vi "GFITS_GetLastHdrs.vi"(10 "ext":string) -> (2 "hdrs":string)   [LabVIEW 2016]
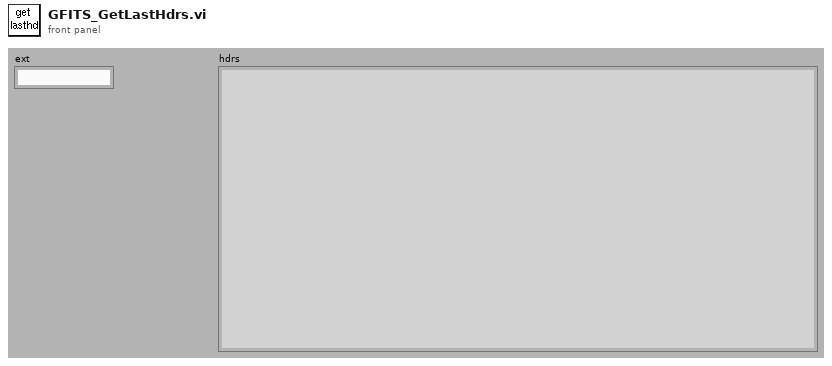
[diagram p1: front panel]
types:
  T1 = enum16{"clear all", "add extension", "add keyword", "get", "clear extension", "done"}
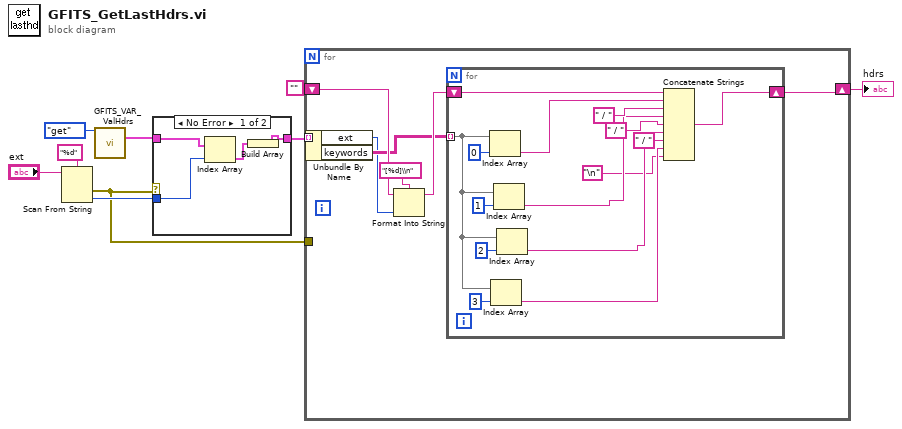
[diagram p0: block diagram]
diagram:
  n1 = Scan From String(format string="%d", input string="ext") -> (error out=w3:errorcluster, output 1=w8:i32)  [unwired: 2 in, 3 out]
  n2 = call "GFITS_VAR_ValHdrs.vi"("action"=T1."get") -> ("last headers"=w1:cluster{"ext":i32, "keywords":string[][]}[])  [unwired: 3 in, 11 out]
  n3 = case shown="No Error" w3 {
    tunnel: w1 -> [w13 w14]
    tunnel: [w11 w14] -> w7
    tunnel: w8 -> [w10 _]
    frame No Error {
      n4 = Index Array(array=w13, index=w10) -> (element=w12:cluster{"ext":i32, "keywords":string[][]})
      n5 = Build Array(w12) -> (w11:cluster{"ext":i32, "keywords":string[][]}[])
    }
    frame Error {
    }
  }
  n6 = for {
    tunnel: w7 -> [w17] mode=indexing
    shift-right: [w18] -> w4
    shift-left: "" -> [w19]
    tunnel: w3 -> [_]
    n7 = Unbundle By Name(w17) -> ("ext"=w15:i32, "keywords"=w16:string[][])
    n8 = Format Into String(format string="[%d]\\n", initial string=w19, w15) -> (resulting string=w20:string)  [unwired: 1 in, 1 out]
    n9 = for {
      tunnel: w16 -> [w33] mode=indexing
      shift-right: [w23] -> w18
      shift-left: w20 -> [w31]
      n10 = Index Array(array=w33, index=0) -> (element=w30:string)
      n11 = Index Array(array=w33, index=3) -> (element=w24:string)
      n12 = Index Array(array=w33, index=1) -> (element=w28:string)
      n13 = Index Array(array=w33, index=2) -> (element=w26:string)
      n14 = Concatenate Strings(w31, w30, " / " ("string"), w28, " / " ("string"), w26, " / " ("string"), w24, "\n") -> (w23:string)
    }
  }
  "hdrs" <- w4
